vi "control.vi"(0 "Camera Device IN":T5, 1 "Image Device IN":cluster{"Image":T4, "errorImage":errorcluster}, 2 "Sound Device IN":T3 {"task ID" format="%.0x"}, 3 "Sound Parameters":cluster{"# samples":u32, "tiempos (ms)":dbl}, 4 "Parametros Maximos":T7, 5 "detla Parametros":T7, 6 "Camara ON?":bool, 7 "Parametros Interferometro/Freq-Volt":T6, 8 "Control?":bool=TRUE, 9 "Reset Control":bool, 10 "Ajuste?":bool=TRUE) -> (14 "Camara Device OUT":T5, 15 "Image Device OUT":cluster{"Image":T4, "errorImage":errorcluster}, 16 "Sound Device OUT":T3 {"task ID" format="%.0x"}, 17 "Contraste":dbl, 18 "Waveform":waveform(dbl), 19 "Señal de Control":dbl[](array[numeric]))   [LabVIEW 2010]
uses:
  <vilib>/vision/Image Controls.llb/IMAQ Image.ctl
  <vilib>/sound2/lvsound2.llb/Sound Output Task ID.ctl
  <vilib>/sound2/lvsound2.llb/Sound Data Format.ctl
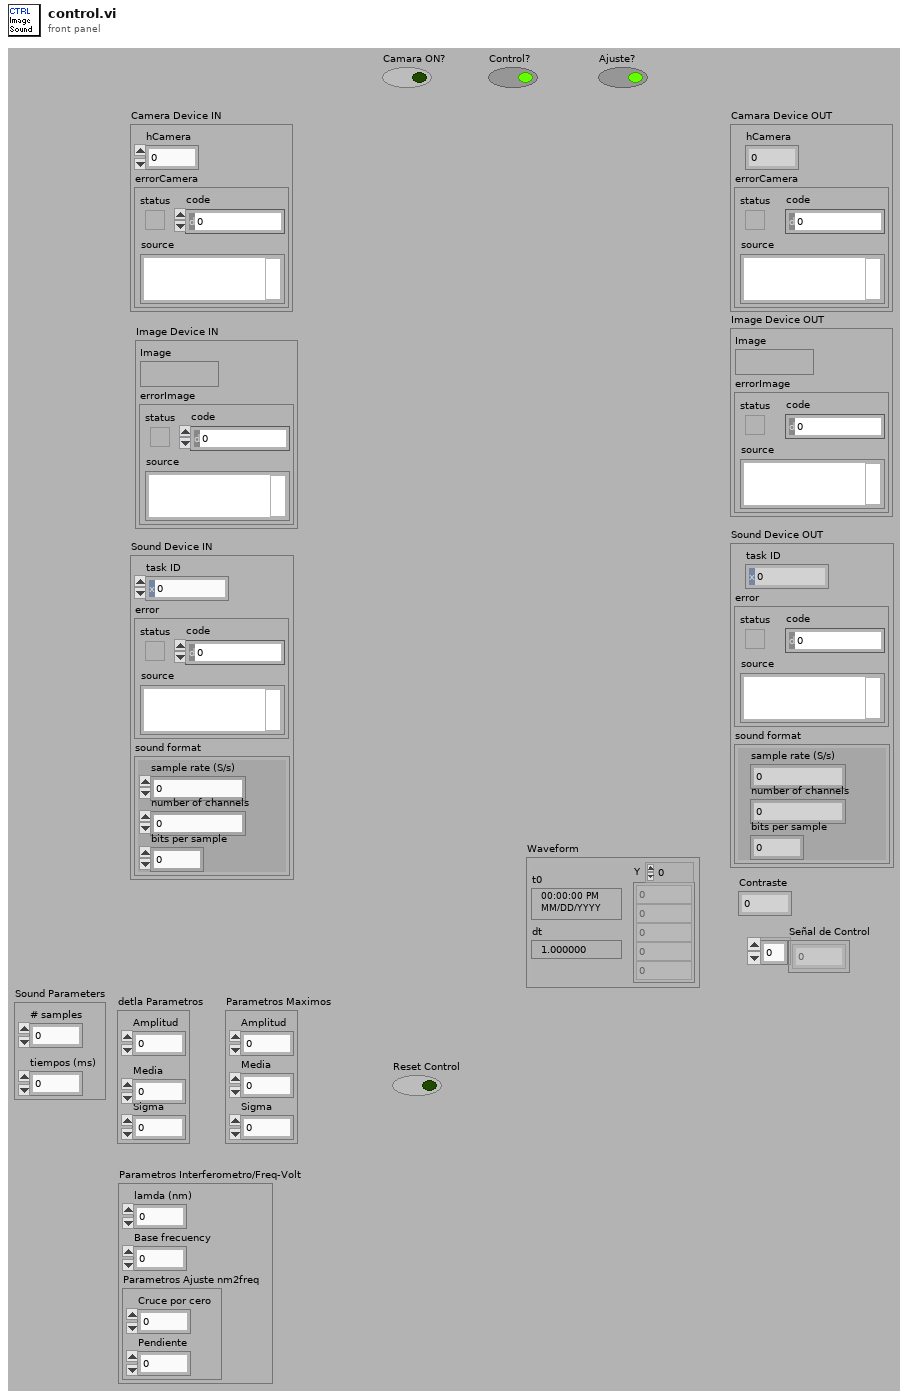
[diagram p1: front panel]
types:
  T1 = typedef "Sound Output Task ID.ctl" = u32
  T2 = typedef "Sound Data Format.ctl" = cluster{"sample rate (S/s)":dbl, "number of channels":i32, "bits per sample":i32}
  T3 = cluster{"task ID":T1, "error":errorcluster, "sound format":T2}
  T4 = typedef "IMAQ Image.ctl" = refnum<image>
  T5 = cluster{"hCamera":u32, "errorCamera":errorcluster}
  T6 = cluster{"lamda (nm)":dbl, "Base frecuency":dbl, "Parametros Ajuste nm2freq":cluster{"Cruce por cero":dbl, "Pendiente":dbl}}
  T7 = cluster{"Amplitud":dbl, "Media":dbl, "Sigma":dbl}
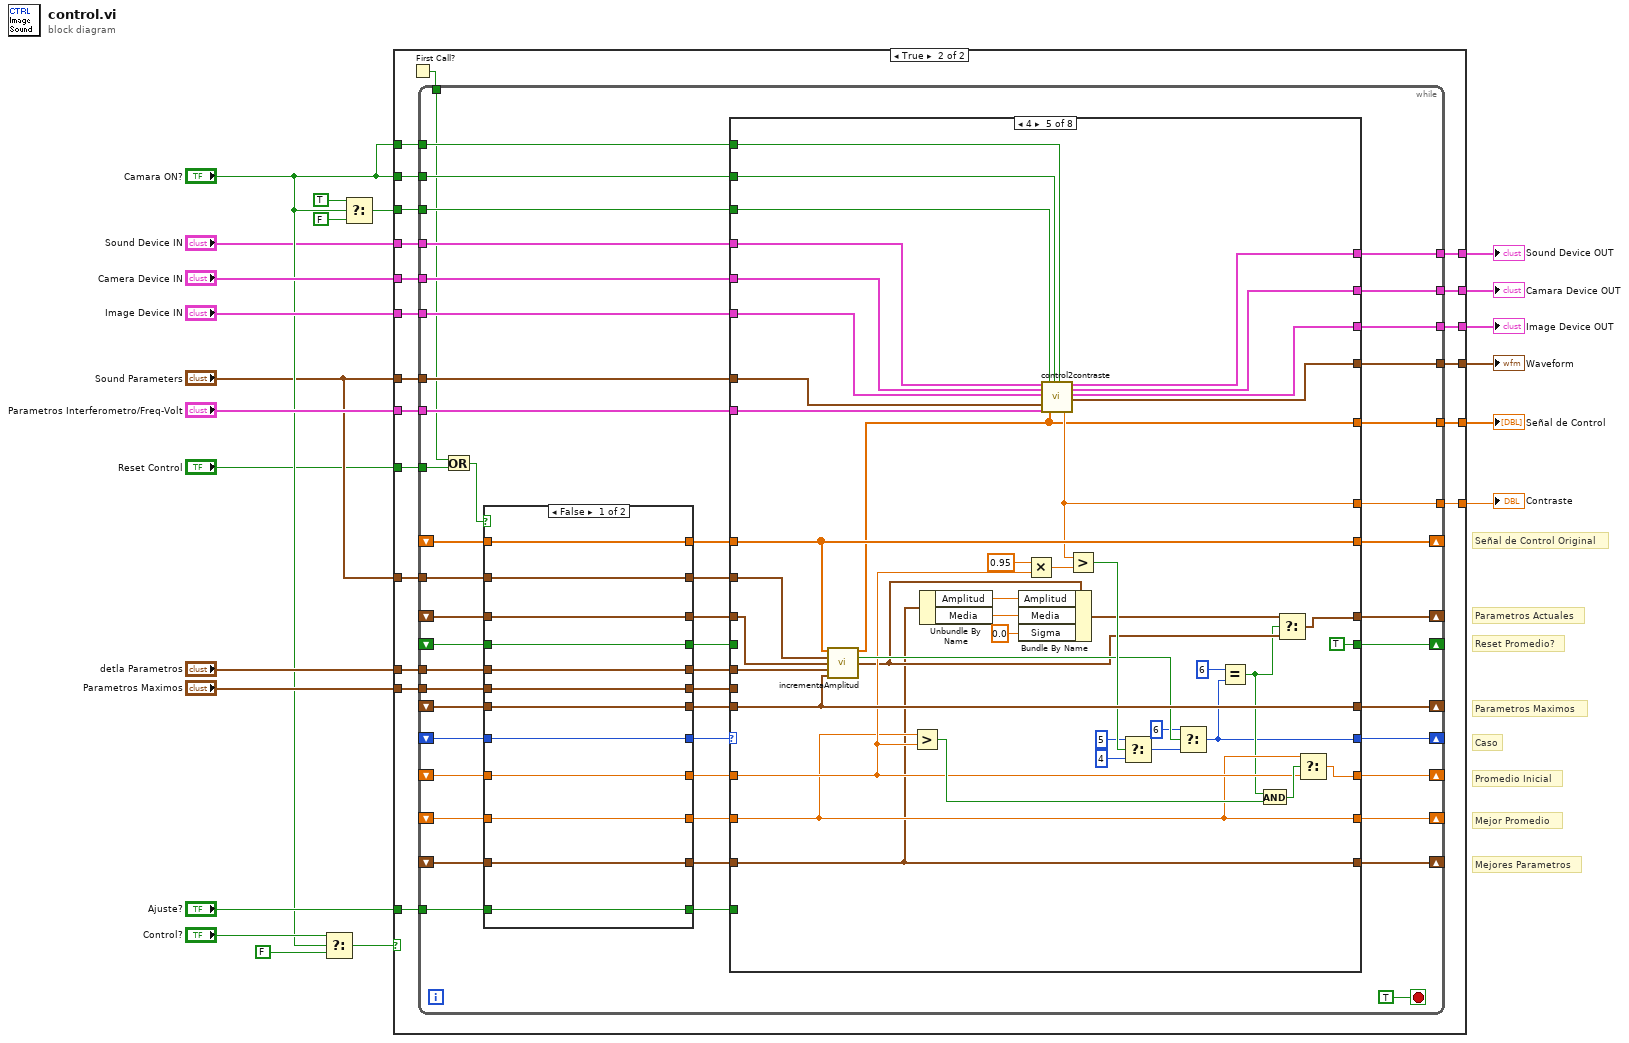
[diagram p0: block diagram]
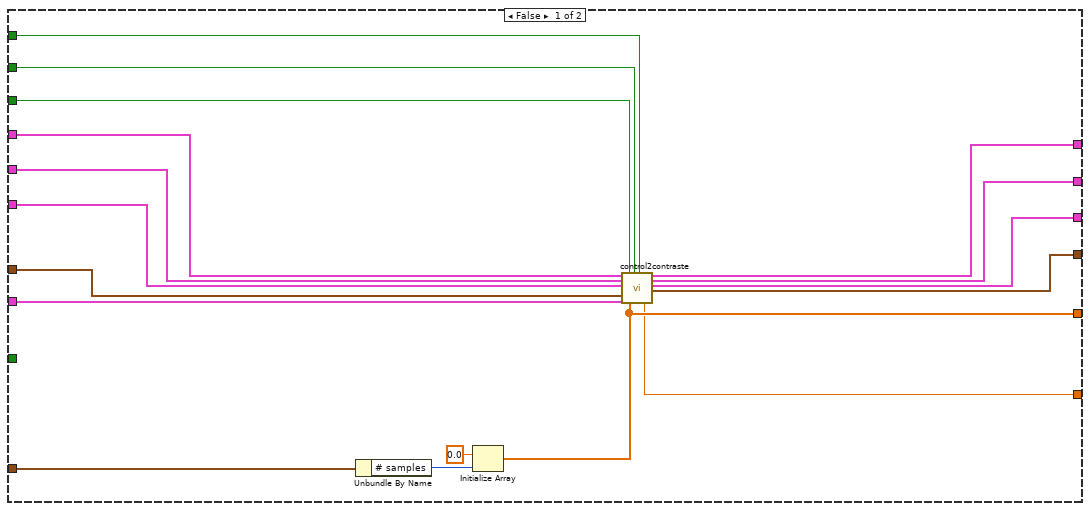
[diagram p2: hidden frame]
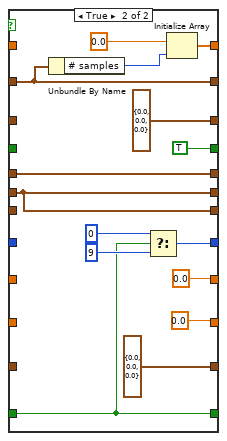
[diagram p3: hidden frame]
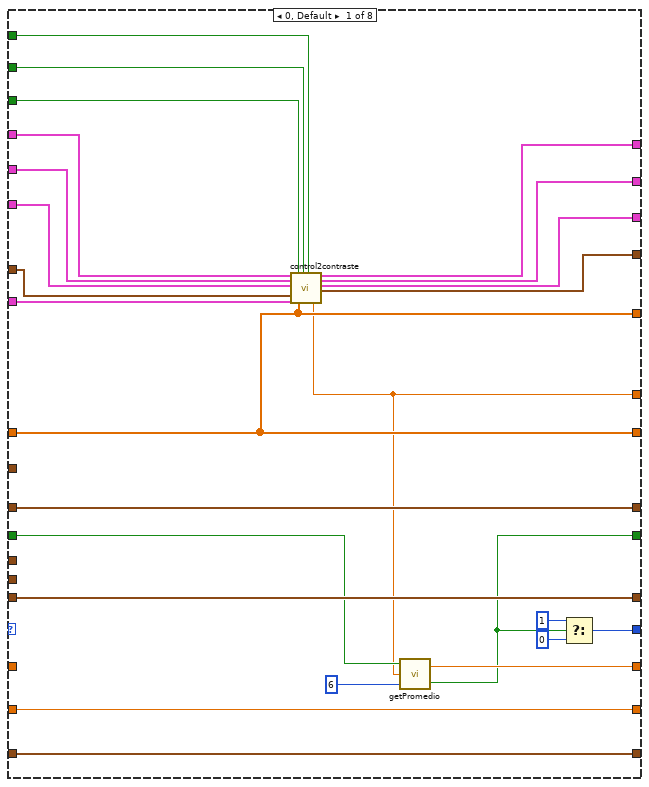
[diagram p4: hidden frame]
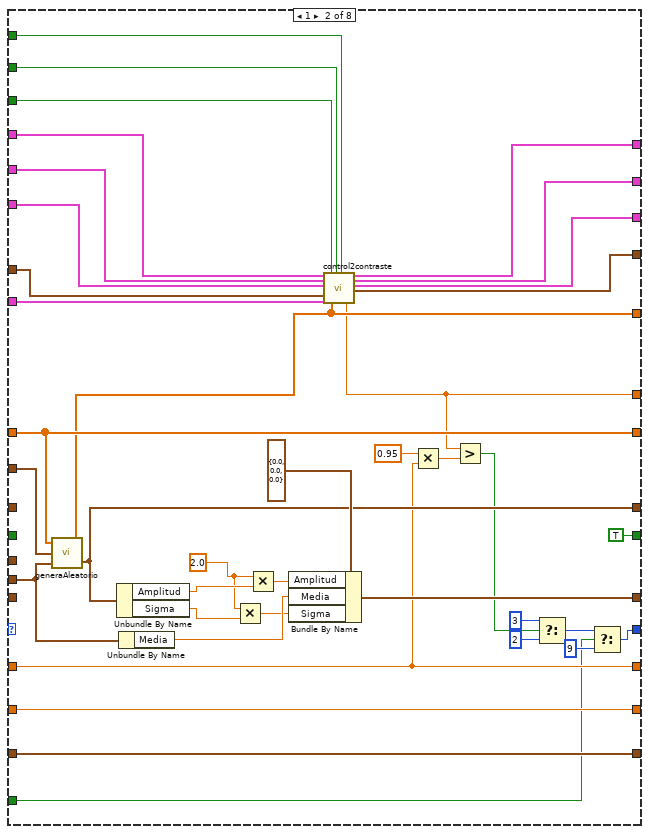
[diagram p5: hidden frame]
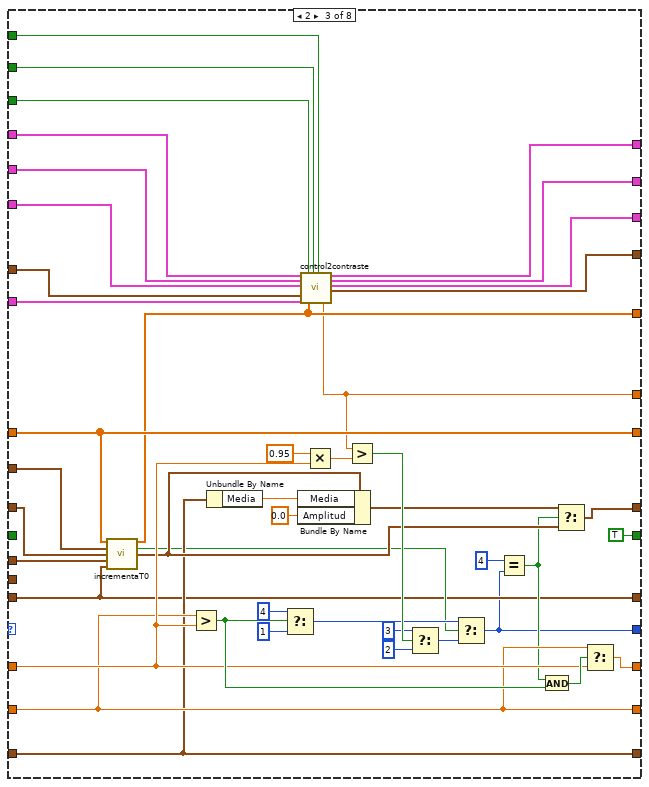
[diagram p6: hidden frame]
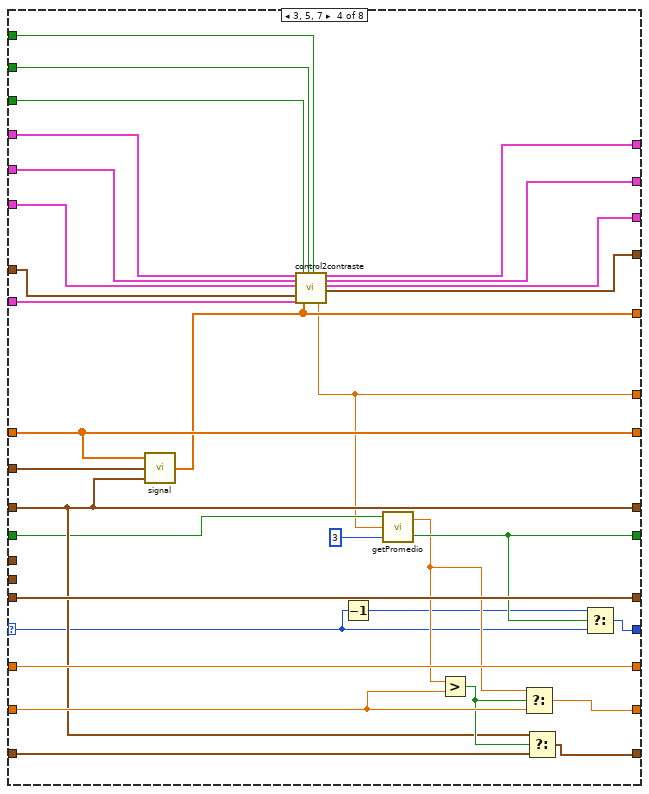
[diagram p7: hidden frame]
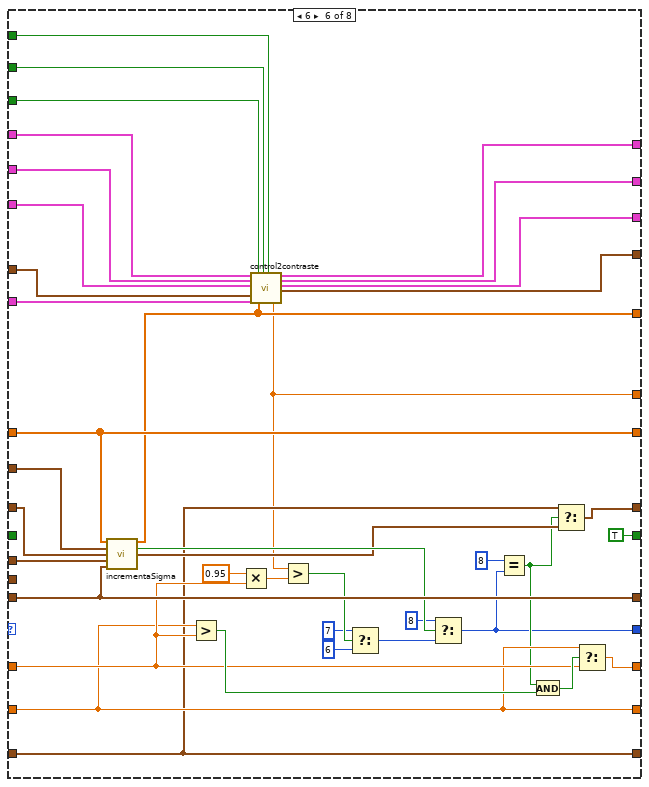
[diagram p8: hidden frame]
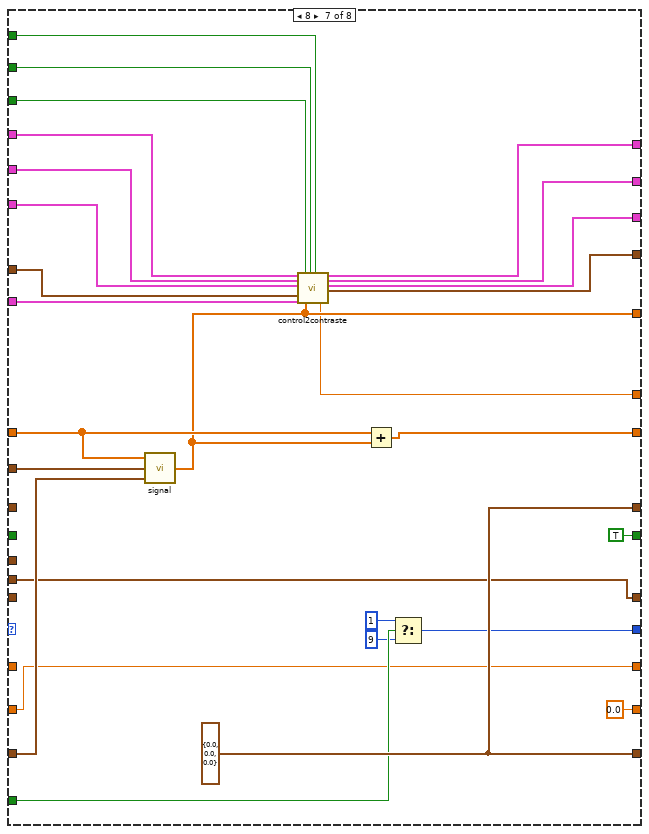
[diagram p9: hidden frame]
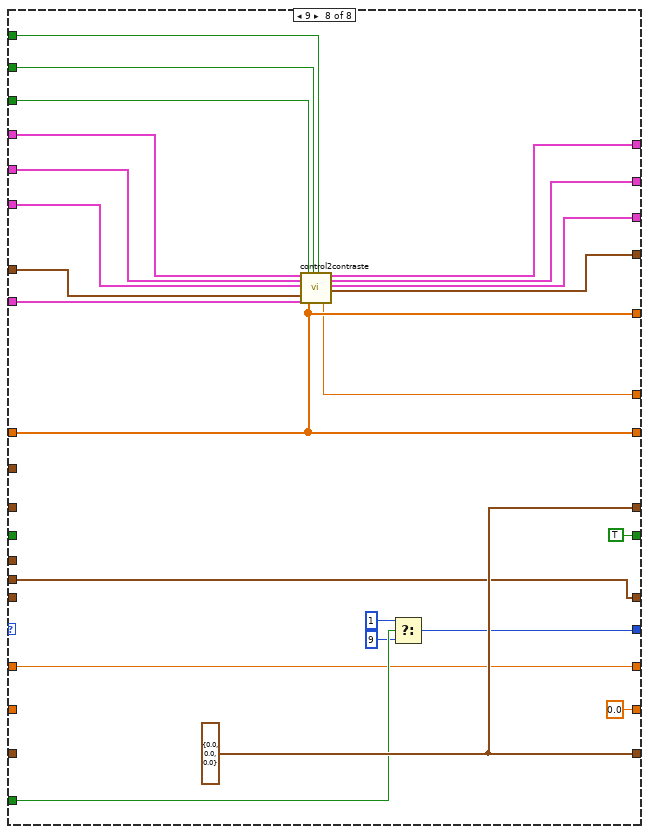
[diagram p10: hidden frame]
diagram:
  # "Reset Promedio?"
  # "Mejores Parametros"
  # "Mejor Promedio"
  # "Señal de Control Original"
  # "Parametros Actuales"
  # "Parametros Maximos"
  # "Caso"
  # "Promedio Inicial"
  n1 = Select(t="Control?", s="Camara ON?", f=FALSE) -> (s? t:f=w8:bool)
  n2 = Select(t=TRUE, s="Camara ON?", f=FALSE) -> (s? t:f=w11:bool)
  n3 = case shown="True" w8 {
    tunnel: "Sound Parameters" -> [w37 w59]
    tunnel: "detla Parametros" -> [_ w58]
    tunnel: "Parametros Maximos" -> [_ w57]
    tunnel: "Ajuste?" -> [_ w55]
    tunnel: [w36 w54] -> w19
    tunnel: [w35 w53] -> w18
    tunnel: "Parametros Interferometro/Freq-Volt" -> [w34 w52]
    tunnel: "Sound Parameters" -> [w33 w51]
    tunnel: "Image Device IN" -> [w32 w50]
    tunnel: "Camera Device IN" -> [w31 w49]
    tunnel: "Sound Device IN" -> [w30 w48]
    tunnel: w11 -> [w29 w47]
    tunnel: "Camara ON?" -> [w28 w46]
    tunnel: "Camara ON?" -> [w27 w45]
    tunnel: [w26 w44] -> w14
    tunnel: [w25 w43] -> w13
    tunnel: [w24 w42] -> w12
    tunnel: [w23 w41] -> w2
    tunnel: "Reset Control" -> [_ w40]
    frame False {
      n4 = Unbundle By Name(w37) -> ("# samples"=w38:u32)
      n5 = Initialize Array(0.0 ("element"), w38) -> (w36:dbl[])
      n6 = call "control2contraste.vi"("Sound Device IN"=w30, "Camera Device IN"=w31, "Image Device IN"=w32, "Sound Parameters"=w33, "Parametros Interferometro/Freq-Volt"=w34, "sound?"=w29, "ControlSignal"=w36, "Streeam?"=w28, "Mostrar?"=w27) -> ("Contraste"=w35:dbl, "Sound Device OUT"=w23:T3, "Camara Device OUT"=w24:T5, "Image Device OUT"=w25:cluster{"Image":T4, "errorImage":errorcluster}, "Waveform"=w26:waveform(dbl))  [unwired: 6 in]
    }
    frame True {
      n7 = First Call?() -> (First Call?: T/F=w56:bool)
      n8 = while {
        shift-right: [w106] -> _
        shift-left: _ -> [w93]
        tunnel: w59 -> [w85]
        shift-right: [w109] -> _
        shift-left: _ -> [w101]
        shift-right: [w108] -> _
        shift-left: _ -> [w95]
        shift-right: [w107] -> _
        shift-left: _ -> [w99]
        shift-right: [w105] -> _
        shift-left: _ -> [w91]
        tunnel: w58 -> [w82]
        shift-right: [w104] -> _
        shift-left: _ -> [w89]
        shift-right: [w103] -> _
        shift-left: _ -> [w87]
        shift-right: [w102] -> _
        shift-left: _ -> [w97]
        tunnel: w55 -> [w84]
        tunnel: w57 -> [w83]
        tunnel: w56 -> [w62]
        tunnel: [w77] -> w54
        tunnel: [w76] -> w53
        tunnel: w52 -> [w75]
        tunnel: w51 -> [w74]
        tunnel: w50 -> [w73]
        tunnel: w49 -> [w72]
        tunnel: w48 -> [w71]
        tunnel: w47 -> [w70]
        tunnel: w46 -> [w69]
        tunnel: w45 -> [w68]
        tunnel: [w67] -> w44
        tunnel: [w66] -> w43
        tunnel: [w65] -> w42
        tunnel: [w64] -> w41
        tunnel: w40 -> [w60]
        stop <- TRUE stop-if-true
        n9 = Or(x=w62, y=w60) -> (x .or. y?=w61:bool)
        n10 = case shown="False" w61 {
          tunnel: w101 -> [w121 _]
          tunnel: [w121 w136] -> w100
          tunnel: [w120 T7 {"Amplitud"=0.0, "Media"=0.0, "Sigma"=0.0} ("Parametros Iniciales")] -> w98
          tunnel: w99 -> [w120 _]
          tunnel: w97 -> [w119 _]
          tunnel: [w119 TRUE] -> w96
          tunnel: w95 -> [w118 _]
          tunnel: [w118 w125] -> w94
          tunnel: w93 -> [w117 _]
          tunnel: [w117 w126] -> w92
          tunnel: w91 -> [w116 _]
          tunnel: [w116 0.0 ("Contraste Promedio")] -> w90
          tunnel: w89 -> [w115 _]
          tunnel: [w115 0.0 ("Contraste Promedio")] -> w88
          tunnel: w87 -> [w114 _]
          tunnel: [w114 T7 {"Amplitud"=0.0, "Media"=0.0, "Sigma"=0.0} ("Parametros Maximos")] -> w86
          tunnel: w85 -> [w113 w122]
          tunnel: w83 -> [w111 w125]
          tunnel: w84 -> [w110 w123]
          tunnel: [w111 w125] -> w81
          tunnel: [w112 w124] -> w80
          tunnel: w82 -> [w112 w124]
          tunnel: [w110 w123] -> w79
          tunnel: [w113 w122] -> w78
          frame False {
          }
          frame True {
            n11 = Unbundle By Name(w122) -> ("# samples"=w134:u32)
            n12 = Select(t=u32 0, s=w123, f=u32 9) -> (s? t:f=w126:u32)
            n13 = Initialize Array(0.0 ("element"), w134) -> (w136:dbl[])
          }
        }
        n14 = case shown="4" w92 {
          selector: w92 -> [_ _ _ w259 _ _ _ _]
          tunnel: w100 -> [w150 w199 w241 w274 w315 w354 w376 w398]
          tunnel: w78 -> [_ w200 w244 w275 w318 w357 w384 _]
          tunnel: w94 -> [w153 _ w219 w265 w314 w353 _ _]
          tunnel: [w150 w199 w241 w274 w315 w354 w375 w398] -> w109
          tunnel: [w153 w198 w219 w265 w314 w353 w372 w400] -> w108
          tunnel: [w154 w196 w227 w264 w302 w341 w381 w406] -> w107
          tunnel: [w160 w162 w202 w272 w276 w319 w373 w401] -> w106
          tunnel: [w155 w185 w233 w271 w308 w347 w374 w399] -> w105
          tunnel: w90 -> [_ w185 w231 w271 w306 w345 _ w399]
          tunnel: [w149 w163 w217 w257 w293 w335 w370 w397] -> w76
          tunnel: [w150 w179 w218 w258 w292 w336 w371 w398] -> w77
          tunnel: w98 -> [w154 _ w243 w264 w317 w356 _ _]
          tunnel: w80 -> [_ _ w242 _ w316 w355 _ _]
          tunnel: [w156 w189 w230 w270 w305 w344 0.0 ("Contraste Promedio") 0.0 ("Contraste Promedio")] -> w104
          tunnel: [w157 w188 w224 w268 w299 w337 w381 w406] -> w103
          tunnel: w86 -> [w157 w188 w224 w266 w299 w337 w383 _]
          tunnel: w88 -> [w156 w189 w230 w269 w305 w344 w374 _]
          tunnel: w96 -> [w151 _ _ w263 _ _ _ _]
          tunnel: [w152 TRUE ("Llego a N?") TRUE ("Llego a N?") w262 TRUE ("Llego a N?") TRUE ("Llego a N?") TRUE ("Llego a N?") TRUE ("Llego a N?")] -> w102
          tunnel: w79 -> [_ w164 _ _ _ _ w379 w404]
          tunnel: w81 -> [_ w180 _ _ _ _ w372 w400]
          tunnel: w75 -> [w148 w178 w216 w256 w291 w334 w369 w396]
          tunnel: w74 -> [w147 w177 w215 w255 w290 w330 w368 w395]
          tunnel: w73 -> [w146 w176 w214 w254 w289 w329 w367 w394]
          tunnel: w72 -> [w145 w175 w213 w253 w288 w328 w366 w393]
          tunnel: w71 -> [w144 w167 w212 w252 w287 w327 w365 w392]
          tunnel: w70 -> [w143 w174 w211 w251 w286 w331 w364 w391]
          tunnel: w69 -> [w142 w173 w210 w250 w285 w332 w363 w390]
          tunnel: w68 -> [w141 w172 w209 w249 w284 w333 w362 w389]
          tunnel: [w140 w171 w208 w248 w283 w326 w361 w388] -> w67
          tunnel: [w139 w169 w207 w247 w282 w325 w360 w387] -> w66
          tunnel: [w138 w170 w206 w246 w281 w324 w359 w386] -> w65
          tunnel: [w137 w168 w205 w245 w280 w323 w358 w385] -> w64
          frame 0, Default {
            n15 = call "control2contraste.vi"("Sound Device IN"=w144, "Camera Device IN"=w145, "Image Device IN"=w146, "Sound Parameters"=w147, "Parametros Interferometro/Freq-Volt"=w148, "sound?"=w143, "ControlSignal"=w150, "Streeam?"=w142, "Mostrar?"=w141) -> ("Contraste"=w149:dbl, "Sound Device OUT"=w137:T3, "Camara Device OUT"=w138:T5, "Image Device OUT"=w139:cluster{"Image":T4, "errorImage":errorcluster}, "Waveform"=w140:waveform(dbl))  [unwired: 6 in]
            n16 = call "getPromedio.vi"("N"=6, "Contraste"=w149, "Reset"=w151) -> ("Llego a N?"=w152:bool, "Contraste Promedio"=w155:dbl)
            n17 = Select(t=u32 1, s=w152, f=u32 0) -> (s? t:f=w160:u32)
          }
          frame 1 {
            w191 = 2.0 ("x")
            n18 = call "generaAleatorio.vi"("Parametros Maximos"=w180, "Sound Parameters"=w200, "Señal de Control IN"=w199) -> ("Parametros Iniciales"=w196:T7, "Out"=w179:dbl[])
            n19 = Unbundle By Name(w196) -> ("Amplitud"=w195:dbl, "Sigma"=w192:dbl)
            n20 = Unbundle By Name(w180) -> ("Media"=w193:dbl)
            n21 = Multiply(x=w191, y=w192) -> (x*y=w190:dbl)
            n22 = Multiply(x=w191, y=w195) -> (x*y=w194:dbl)
            n23 = Bundle By Name(cluster=T7 {"Amplitud"=0.0, "Media"=0.0, "Sigma"=0.0} ("Parametros Iniciales"), "Amplitud"=w194, "Media"=w193, "Sigma"=w190) -> (w198:T7)
            n24 = call "control2contraste.vi"("Sound Device IN"=w167, "Camera Device IN"=w175, "Image Device IN"=w176, "Sound Parameters"=w177, "Parametros Interferometro/Freq-Volt"=w178, "sound?"=w174, "ControlSignal"=w179, "Streeam?"=w173, "Mostrar?"=w172) -> ("Contraste"=w163:dbl, "Sound Device OUT"=w168:T3, "Camara Device OUT"=w170:T5, "Image Device OUT"=w169:cluster{"Image":T4, "errorImage":errorcluster}, "Waveform"=w171:waveform(dbl))  [unwired: 6 in]
            n25 = Multiply(x=0.95, y=w185) -> (x*y=w187:dbl)
            n26 = Greater?(x=w163, y=w187) -> (0:w184:bool)
            n27 = Select(t=u32 3, s=w184, f=u32 2) -> (s? t:f=w165:u32)
            n28 = Select(t=w165, s=w164, f=u32 9) -> (s? t:f=w162:u32)
          }
          frame 2 {
            n29 = call "incrementaT0.vi"("Señal de Control IN"=w241, "Sound Parameters"=w244, "Parametros Actuales IN"=w243, "detla Parametros"=w242, "Parametros Maximos"=w219) -> ("Out"=w218:dbl[], "Tope?"=w221:bool, "Parametros Actuales OUT"=w225:T7)  [unwired: 8 in]
            n30 = Greater?(x=w230, y=w231) -> (0:w234:bool)
            n31 = Unbundle By Name(w224) -> ("Media"=w223:dbl)
            n32 = Select(t=u32 4, s=w234, f=u32 1) -> (s? t:f=w235:u32)
            n33 = Bundle By Name(cluster=w225, "Media"=w223, "Amplitud"=0.0) -> (w226:T7)
            n34 = call "control2contraste.vi"("Sound Device IN"=w212, "Camera Device IN"=w213, "Image Device IN"=w214, "Sound Parameters"=w215, "Parametros Interferometro/Freq-Volt"=w216, "sound?"=w211, "ControlSignal"=w218, "Streeam?"=w210, "Mostrar?"=w209) -> ("Contraste"=w217:dbl, "Sound Device OUT"=w205:T3, "Camara Device OUT"=w206:T5, "Image Device OUT"=w207:cluster{"Image":T4, "errorImage":errorcluster}, "Waveform"=w208:waveform(dbl))  [unwired: 6 in]
            n35 = Multiply(x=0.95, y=w231) -> (x*y=w240:dbl)
            n36 = Greater?(x=w217, y=w240) -> (0:w238:bool)
            n37 = Select(t=u32 3, s=w238, f=u32 2) -> (s? t:f=w201:u32)
            n38 = Select(t=w235, s=w221, f=w201) -> (s? t:f=w202:u32)
            n39 = Equal?(x=u32 4, y=w202) -> (x = y?=w220:bool)
            n40 = And(x=w220, y=w234) -> (x .and. y?=w232:bool)
            n41 = Select(t=w226, s=w220, f=w225) -> (s? t:f=w227:T7)
            n42 = Select(t=w230, s=w232, f=w231) -> (s? t:f=w233:dbl)
          }
          frame 3, 5, 7 {
            n43 = call "signal.vi"("Parametros Actuales IN"=w264, "Sound Parameters"=w275, "Señal de Control IN"=w274) -> ("Out"=w258:dbl[])
            n44 = call "control2contraste.vi"("Sound Device IN"=w252, "Camera Device IN"=w253, "Image Device IN"=w254, "Sound Parameters"=w255, "Parametros Interferometro/Freq-Volt"=w256, "sound?"=w251, "ControlSignal"=w258, "Streeam?"=w250, "Mostrar?"=w249) -> ("Contraste"=w257:dbl, "Sound Device OUT"=w245:T3, "Camara Device OUT"=w246:T5, "Image Device OUT"=w247:cluster{"Image":T4, "errorImage":errorcluster}, "Waveform"=w248:waveform(dbl))  [unwired: 6 in]
            n45 = Decrement(x=w259) -> (x-1=w260:u32)
            n46 = call "getPromedio.vi"("N"=3, "Contraste"=w257, "Reset"=w263) -> ("Llego a N?"=w262:bool, "Contraste Promedio"=w261:dbl)
            n47 = Greater?(x=w261, y=w269) -> (0:w267:bool)
            n48 = Select(t=w261, s=w267, f=w269) -> (s? t:f=w270:dbl)
            n49 = Select(t=w264, s=w267, f=w266) -> (s? t:f=w268:T7)
            n50 = Select(t=w260, s=w262, f=w259) -> (s? t:f=w272:u32)
          }
          frame 4 {
            n51 = call "incrementaAmplitud.vi"("Señal de Control IN"=w315, "Sound Parameters"=w318, "Parametros Actuales IN"=w317, "detla Parametros"=w316, "Parametros Maximos"=w314) -> ("Out"=w292:dbl[], "Tope?"=w310:bool, "Parametros Actuales OUT"=w300:T7)  [unwired: 8 in]
            n52 = Greater?(x=w305, y=w306) -> (0:w309:bool)
            n53 = Unbundle By Name(w299) -> ("Amplitud"=w298:dbl, "Media"=w296:dbl)
            n54 = Bundle By Name(cluster=w300, "Amplitud"=w298, "Media"=w296, "Sigma"=0.0 ("Amplitud")) -> (w301:T7)
            n55 = Multiply(x=0.95, y=w306) -> (x*y=w313:dbl)
            n56 = call "control2contraste.vi"("Sound Device IN"=w287, "Camera Device IN"=w288, "Image Device IN"=w289, "Sound Parameters"=w290, "Parametros Interferometro/Freq-Volt"=w291, "sound?"=w286, "ControlSignal"=w292, "Streeam?"=w285, "Mostrar?"=w284) -> ("Contraste"=w293:dbl, "Sound Device OUT"=w280:T3, "Camara Device OUT"=w281:T5, "Image Device OUT"=w282:cluster{"Image":T4, "errorImage":errorcluster}, "Waveform"=w283:waveform(dbl))  [unwired: 6 in]
            n57 = Greater?(x=w293, y=w313) -> (0:w311:bool)
            n58 = Select(t=u32 5, s=w311, f=u32 4) -> (s? t:f=w277:u32)
            n59 = Select(t=u32 6, s=w310, f=w277) -> (s? t:f=w276:u32)
            n60 = Equal?(x=u32 6, y=w276) -> (x = y?=w294:bool)
            n61 = And(x=w294, y=w309) -> (x .and. y?=w307:bool)
            n62 = Select(t=w301, s=w294, f=w300) -> (s? t:f=w302:T7)
            n63 = Select(t=w305, s=w307, f=w306) -> (s? t:f=w308:dbl)
          }
          frame 6 {
            n64 = call "incrementaSigma.vi"("Señal de Control IN"=w354, "Sound Parameters"=w357, "Parametros Actuales IN"=w356, "detla Parametros"=w355, "Parametros Maximos"=w353) -> ("Out"=w336:dbl[], "Tope?"=w349:bool, "Parametros Actuales OUT"=w340:T7)  [unwired: 8 in]
            n65 = Greater?(x=w344, y=w345) -> (0:w348:bool)
            n66 = Multiply(x=0.95, y=w345) -> (x*y=w352:dbl)
            n67 = call "control2contraste.vi"("Sound Device IN"=w327, "Camera Device IN"=w328, "Image Device IN"=w329, "Sound Parameters"=w330, "Parametros Interferometro/Freq-Volt"=w334, "sound?"=w331, "ControlSignal"=w336, "Streeam?"=w332, "Mostrar?"=w333) -> ("Contraste"=w335:dbl, "Sound Device OUT"=w323:T3, "Camara Device OUT"=w324:T5, "Image Device OUT"=w325:cluster{"Image":T4, "errorImage":errorcluster}, "Waveform"=w326:waveform(dbl))  [unwired: 6 in]
            n68 = Greater?(x=w335, y=w352) -> (0:w350:bool)
            n69 = Select(t=u32 7, s=w350, f=u32 6) -> (s? t:f=w320:u32)
            n70 = Select(t=u32 8, s=w349, f=w320) -> (s? t:f=w319:u32)
            n71 = Equal?(x=u32 8, y=w319) -> (x = y?=w338:bool)
            n72 = And(x=w338, y=w348) -> (x .and. y?=w346:bool)
            n73 = Select(t=w337, s=w338, f=w340) -> (s? t:f=w341:T7)
            n74 = Select(t=w344, s=w346, f=w345) -> (s? t:f=w347:dbl)
          }
          frame 8 {
            w381 = T7 {"Amplitud"=0.0, "Media"=0.0, "Sigma"=0.0} ("Parametros Maximos")
            n75 = call "signal.vi"("Parametros Actuales IN"=w383, "Sound Parameters"=w384, "Señal de Control IN"=w376) -> ("Out"=w371:dbl[])
            n76 = call "control2contraste.vi"("Sound Device IN"=w365, "Camera Device IN"=w366, "Image Device IN"=w367, "Sound Parameters"=w368, "Parametros Interferometro/Freq-Volt"=w369, "sound?"=w364, "ControlSignal"=w371, "Streeam?"=w363, "Mostrar?"=w362) -> ("Contraste"=w370:dbl, "Sound Device OUT"=w358:T3, "Camara Device OUT"=w359:T5, "Image Device OUT"=w360:cluster{"Image":T4, "errorImage":errorcluster}, "Waveform"=w361:waveform(dbl))  [unwired: 6 in]
            n77 = Add(x=w376, y=w371) -> (x+y=w375:dbl[])
            n78 = Select(t=u32 1, s=w379, f=u32 9) -> (s? t:f=w373:u32)
          }
          frame 9 {
            w406 = T7 {"Amplitud"=0.0, "Media"=0.0, "Sigma"=0.0} ("Parametros Maximos")
            n79 = call "control2contraste.vi"("Sound Device IN"=w392, "Camera Device IN"=w393, "Image Device IN"=w394, "Sound Parameters"=w395, "Parametros Interferometro/Freq-Volt"=w396, "sound?"=w391, "ControlSignal"=w398, "Streeam?"=w390, "Mostrar?"=w389) -> ("Contraste"=w397:dbl, "Sound Device OUT"=w385:T3, "Camara Device OUT"=w386:T5, "Image Device OUT"=w387:cluster{"Image":T4, "errorImage":errorcluster}, "Waveform"=w388:waveform(dbl))  [unwired: 6 in]
            n80 = Select(t=u32 1, s=w404, f=u32 9) -> (s? t:f=w401:u32)
          }
        }
      }
    }
  }
  "Señal de Control" <- w19
  "Contraste" <- w18
  "Camara Device OUT" <- w12
  "Image Device OUT" <- w13
  "Waveform" <- w14
  "Sound Device OUT" <- w2
